vi "5b - DSTP read.vi"() -> ()   [LabVIEW 2010]
panel:
  in  "stop":bool
  in  "numbers":dbl
  out "Waveform Chart":dbl(graph)
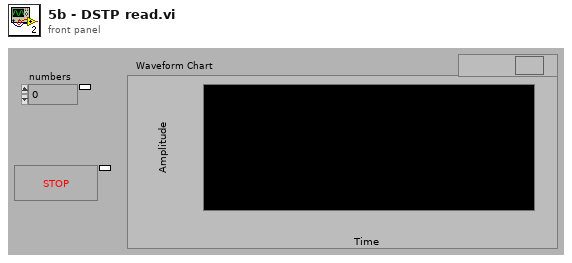
[diagram p1: front panel]
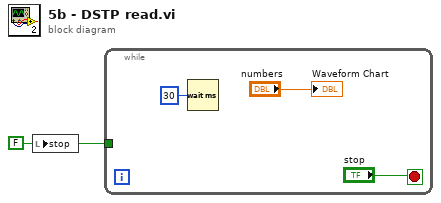
[diagram p0: block diagram]
diagram:
  w1 = FALSE ("stop")
  n1 = local write "stop"(w1) -> ()
  n2 = while {
    tunnel: w1 -> [_]
    stop <- "stop" stop-if-true
    n3 = Wait (ms)(milliseconds to wait=u32 30) -> ()  [unwired: 1 out]
    "Waveform Chart" <- "numbers"
  }
